vi "Archive.vi"(8 "error in (no error)":errorcluster, 11 "System Configuration":T1) -> (0 "error out":errorcluster)   [LabVIEW 2024]
doc: "Archives data."
uses:
  Controls/Server/System Configuration.ctl
  Controls/Server/Subsystem Configuration.ctl
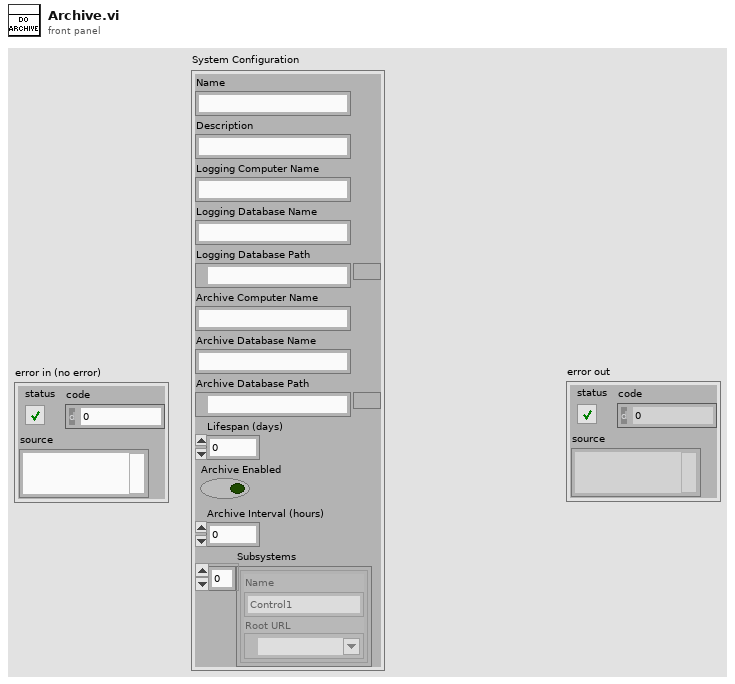
[diagram p1: front panel]
types:
  T1 = typedef "System Configuration.ctl" = cluster{"Name":string, "Description":string, "Logging Computer Name":string, "Logging Database Name":string, "Logging Database Path":path, "Archive Computer Name":string, "Archive Database Name":string, "Archive Database Path":path, "Lifespan (days)":u32, "Archive Enabled":bool, "Archive Interval (hours)":u32, "Subsystems":T2[]}
  T2 = typedef "Subsystem Configuration.ctl" = cluster{"Name":string, "Root URL":refnum<k21>}
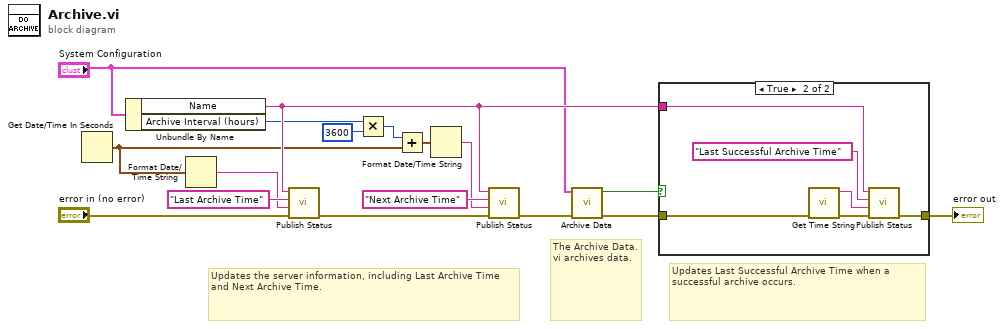
[diagram p0: block diagram]
diagram:
  # "Updates Last Successful Archive Time when a successful archive occurs."
  # "The Archive Data.vi archives data."
  # "Updates the server information, including Last Archive Time and Next Archive Time."
  n1 = Get Date/Time In Seconds() -> (seconds since 1Jan1904=w8:timestamp)
  n2 = Unbundle By Name("System Configuration") -> ("Name"=w14:string, "Archive Interval (hours)"=w7:u32)
  n3 = Format Date/Time String(seconds (now)=w8) -> (date/time string=w11:string)  [unwired: 2 in]
  n4 = call "Publish Status.vi"("error in (no error)"="error in (no error)", "Value"=w11, "Parameter"="Last Archive Time", "System Name"=w14) -> ("error out"=w4:errorcluster)  [unwired: 7 in]
  n5 = Multiply(x=w7, y=3600) -> (x*y=w9:u32)
  n6 = Add(x=w9, y=w8) -> (x+y=w12:timestamp)
  n7 = Format Date/Time String(seconds (now)=w12) -> (date/time string=w10:string)  [unwired: 2 in]
  n8 = call "Publish Status.vi"("error in (no error)"=w4, "Value"=w10, "Parameter"="Next Archive Time", "System Name"=w14) -> ("error out"=w3:errorcluster)  [unwired: 7 in]
  n9 = call "Archive Data.vi"("error in (no error)"=w3, "System Configuration"="System Configuration") -> ("error out"=w5:errorcluster, "Succeed?"=w6:bool)  [unwired: 8 in]
  n10 = case shown="True" w6 {
    tunnel: w14 -> [_ w20]
    tunnel: [w18 w21] -> w1
    tunnel: w5 -> [w18 w19]
    frame False {
    }
    frame True {
      n11 = call "Get Time String.vi"("error in (no error)"=w19) -> ("error out"=w22:errorcluster, "Time String"=w23:string)  [unwired: 9 in]
      n12 = call "Publish Status.vi"("error in (no error)"=w22, "Value"=w23, "Parameter"="Last Successful Archive Time", "System Name"=w20) -> ("error out"=w21:errorcluster)  [unwired: 7 in]
    }
  }
  "error out" <- w1
